vi "StateMachineRealTimeTrackerVI.vi"() -> ()   [LabVIEW 2015]
uses:
  StateMachineObjectTracker/qsm/type defs/mode buttons.ctl
  StateMachineObjectTracker/qsm/type defs/state.ctl
  StateMachineObjectTracker/qsm/type defs/data.ctl
  StateMachineObjectTracker/qsm/type defs/task.ctl
  <vilib>/myRIO/Instrument Drivers/Onboard IO/DIO/typedefs/DIO Reference.ctl
  <vilib>/myRIO/Common/Instrument Driver Framework/Utilities/typedefs/myRIO Generic Hardware Reference.ctl
  <vilib>/myRIO/Common/Instrument Driver Framework/Utilities/typedefs/Hardware Version Enum.ctl
  <vilib>/myRIO/Common/Instrument Driver Framework/Utilities/typedefs/myRIO v1.0 Reference.ctl
  <vilib>/myRIO/Common/Instrument Driver Framework/Utilities/typedefs/Generic FPGA Reference.ctl
  <vilib>/myRIO/Common/Instrument Driver Framework/myRIO v1.0/DIO/typedefs/DIO Channels List.ctl
  <vilib>/myRIO/Common/Instrument Driver Framework/myRIO v1.0/DIO/typedefs/DIO Channels Enum.ctl
  <vilib>/userdefined/High Color/nirio_resource_hc.ctl
  <vilib>/myRIO/Common/Instrument Driver Framework/Utilities/vis/Is FPGA Ref Available.vi
  <vilib>/myRIO/Common/Instrument Driver Framework/myRIO v1.0/DIO/vis/myRIO v1.1 Open DIO.vi
  <vilib>/myRIO/Instrument Drivers/Onboard IO/DIO/vis/Write.vi
  <vilib>/myRIO/Common/Instrument Driver Framework/Utilities/vis/Validate Channels.vi
  <vilib>/myRIO/Common/Instrument Driver Framework/myRIO v1.0/DIO/vis/myRIO v1.0 Reserve DIO.vi
  <vilib>/myRIO/Common/Instrument Driver Framework/myRIO v1.0/Resource Manager/vis/myRIO v1.0 Reserve Channel List.vi
  <vilib>/myRIO/Common/Instrument Driver Framework/myRIO v1.0/DIO/vis/myRIO v1.0 Build MUX Configuration DIO.vi
  <vilib>/myRIO/Common/Instrument Driver Framework/myRIO v1.0/Resource Manager/vis/myRIO v1.0 Reserve Channel.vi
  <vilib>/myRIO/Common/Instrument Driver Framework/myRIO v1.0/Resource Manager/vis/myRIO v1.0 Unreserve Channel.vi
  <vilib>/myRIO/Common/Instrument Driver Framework/myRIO v1.0/Resource Manager/vis/myRIO v1.0 Create Configuration List.vi
  <vilib>/myRIO/Common/Instrument Driver Framework/myRIO v1.0/Resource Manager/vis/myRIO v1.0 Build Mutex Name.vi
  <vilib>/Utility/VariantDataType/GetNumericInfo.vi
  <vilib>/Utility/error.llb/Error Cluster From Error Code.vi
  <vilib>/myRIO/Common/Instrument Driver Framework/myRIO v1.0/myRIO v1.1 Open.vi
  <vilib>/myRIO/Common/Instrument Driver Framework/Utilities/vis/IO Manager.vi
  <vilib>/myRIO/Common/Instrument Driver Framework/Utilities/vis/Configuration Manager.vi
  <vilib>/myRIO/Common/Instrument Driver Framework/myRIO v1.0/Resource Manager/vis/myRIO v1.0 Configure IO.vi
  <vilib>/myRIO/Common/Instrument Driver Framework/myRIO v1.0/myRIO v1.0 Close.vi
  <vilib>/myRIO/Common/Instrument Driver Framework/myRIO v1.0/DIO/vis/myRIO v1.0 Write DIO.vi
  <vilib>/myRIO/Express VI/Onboard Devices/LED/LED Express VI.xnode
  <vilib>/myRIO/Instrument Drivers/Onboard IO/DIO/vis/myRIO DIO Open.xnode
  <vilib>/myRIO/Instrument Drivers/Onboard IO/DIO/DIO.lvlib
panel:
  in  "Stop":bool
  in  "mode buttons":T1
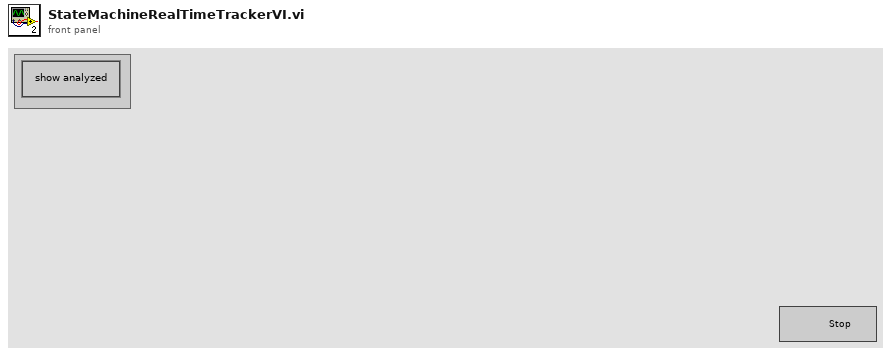
[diagram p1: front panel]
types:
  T1 = typedef "mode buttons.ctl" = cluster{"show analyzed":bool}
  T2 = typedef "data.ctl" = cluster{"Status Test":string}
  T3 = typedef "state.ctl" = enum16{"(qsm) schedule", "(qsm) initialize", "(qsm) release", "(qsm) clean up", "(qsm) shutdown", "(myRIO) initialize", "(myRIO) clean up", "(myRIO) update ports", "(image) get", "(image) analyze", "(image) overlay", "(image) show", "save image", "state A", "state B", "state C", "state D", "state E", "state F", "state G", "state H"}
  T4 = typedef "DIO.lvlib/DIO Reference.ctl" = cluster{"myRIO Reference":T5, "DIO Channels List":T9}
  T5 = typedef "myRIO Generic Hardware Reference.ctl" = cluster{"myRIO Model":T6, "myRIO Hardware Reference":T7}
  T6 = typedef "Hardware Version Enum.ctl" = enum16{"Unknown", "myRIO-1900", "myRIO-1950", "roboRIO"}
  T7 = typedef "myRIO v1.0 Reference.ctl" = cluster{"Generic FPGA Reference":T8, "Allow multiple opens":bool}
  T8 = typedef "Generic FPGA Reference.ctl" = refnum<k20>
  T9 = typedef "DIO Channels List.ctl" = T10[]
  T10 = typedef "DIO Channels Enum.ctl" = enum16{"Not Connected", "C/DIO0", "C/DIO1", "C/DIO2", "C/DIO3", "C/DIO4", "C/DIO5", "C/DIO6", "C/DIO7", "A/DIO0", "A/DIO1", "A/DIO2", "A/DIO3", "A/DIO4", "A/DIO5", "A/DIO6", "A/DIO7", "A/DIO8", "A/DIO9", "A/DIO10", "A/DIO11", "A/DIO12", "A/DIO13", "A/DIO14", "A/DIO15", "B/DIO0", "B/DIO1", "B/DIO2", "B/DIO3", "B/DIO4", "B/DIO5", "B/DIO6", "B/DIO7", "B/DIO8", "B/DIO9", "B/DIO10", "B/DIO11", "B/DIO12", "B/DIO13", "B/DIO14", "B/DIO15", "LED0", "LED1", "LED2", "LED3", "Button0", "DIO/DIO0", "DIO/DIO1", "DIO/DIO2", "DIO/DIO3", "DIO/DIO4", "DIO/DIO5", "DIO/DIO6", "DIO/DIO7", "DIO/DIO8", "DIO/DIO9", "SPI/CS0", "SPI/CS1", "SPI/CS2", "SPI/CS3", "LED RADIO (Green)", "LED RADIO (Red)", "LED COMM (Green)", "LED COMM (Red)", "LED MODE (Green)", "LED MODE (Red)"}
  T11 = typedef "nirio_resource_hc.ctl" = tag
  T12 = typedef "task.ctl" = T3[]
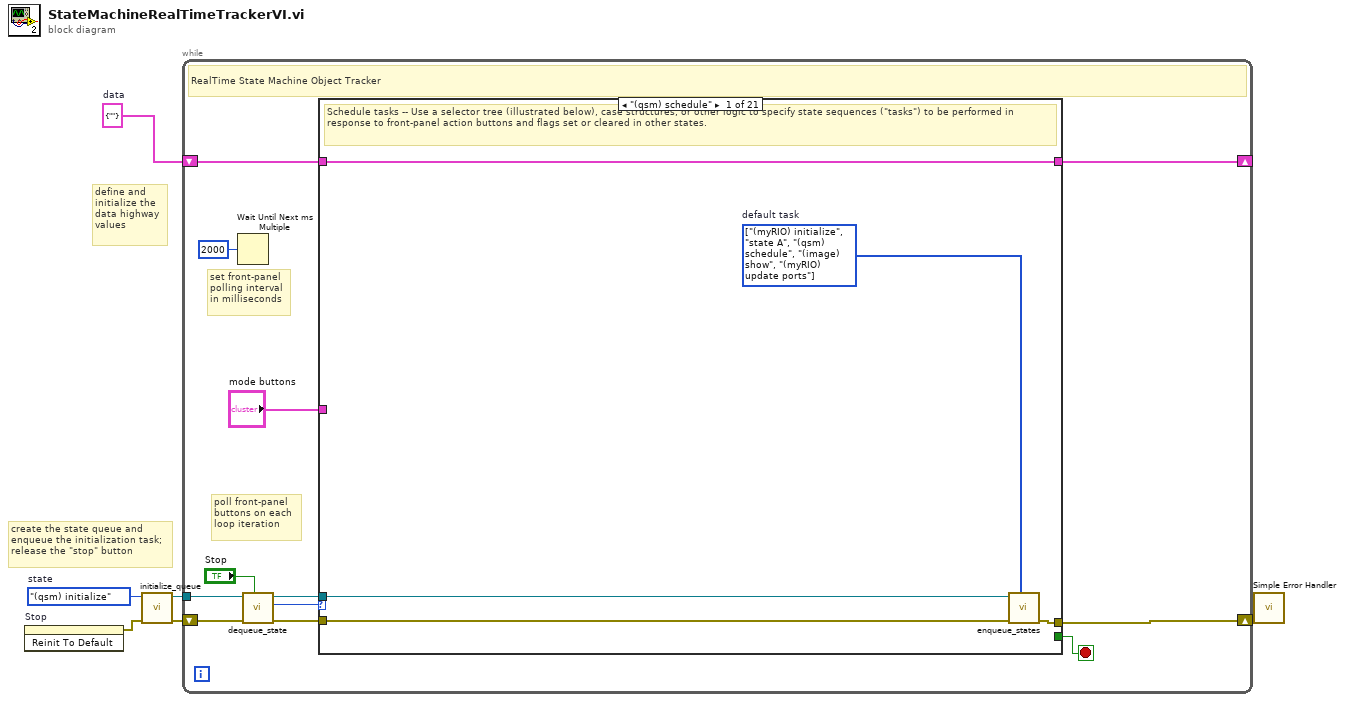
[diagram p0: block diagram]
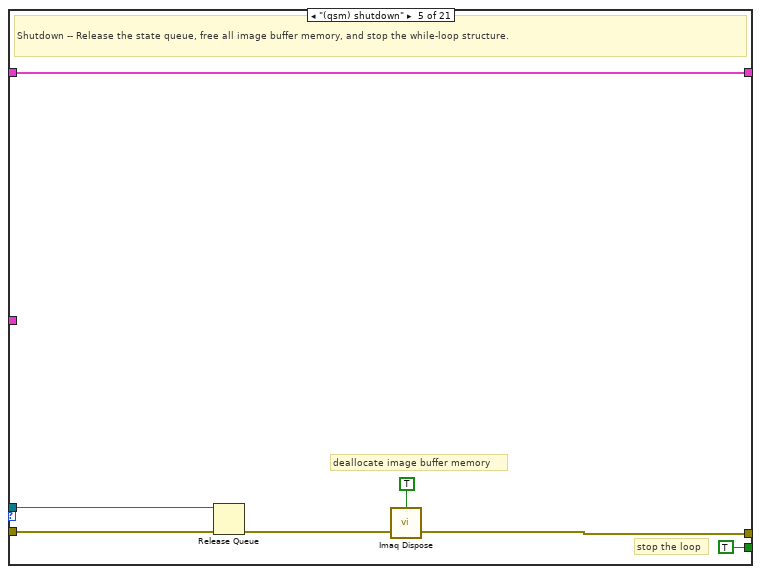
[diagram p5: hidden frame]
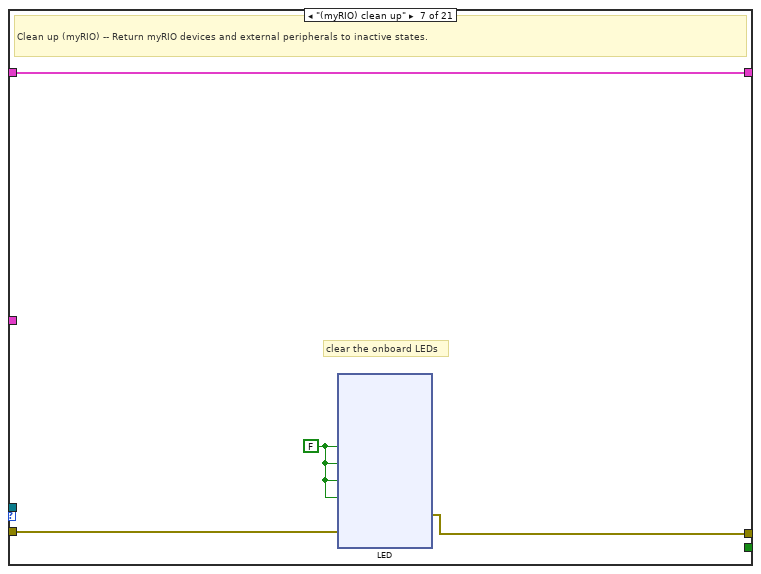
[diagram p7: hidden frame]
diagram:
  w5 = T2 {"Status Test"=""}  # data
  w1 = state."(qsm) initialize"  # state
  # "define and \ninitialize the \ndata highway\nvalues"
  # "create the state queue and\nenqueue the initialization task;\nrelease the \"stop\" button"
  n1 = invoke on="Stop" class="Bool" method="Reinit To Default"() -> (error out=w2:errorcluster)  [unwired: 3 in, 2 out]
  n2 = call "initialize_queue.vi"("error in (no error)"=w2, "state"=w1) -> ("error out"=w4:errorcluster, "queue out"=w3:refnum<queue>)  [unwired: 8 in]
  n3 = while {
    shift-right: [w18] -> w6
    shift-left: w4 -> [w12]
    tunnel: w3 -> [w13]
    shift-right: [w16] -> _
    shift-left: w5 -> [w17]
    stop <- w15 stop-if-true
    # "set front-panel\npolling interval\nin milliseconds"
    # "poll front-panel\nbuttons on each\nloop iteration"
    # "RealTime State Machine Object Tracker"
    n4 = Wait Until Next ms Multiple(millisecond multiple=u32 2000) -> ()  [unwired: 1 out]
    n5 = call "dequeue_state.vi"("stop"="Stop", "error in (no error)"=w12, "queue in"=w13) -> ("error out"=w14:errorcluster, "state"=w7:T3, "queue out"=w10:refnum<queue>)  [unwired: 6 in]
    n6 = case shown="\"(qsm) schedule\"" w7 {
      tunnel: w14 -> [w20 w25 w26 w29 w35 w37 w40 w82 w83 w85 w87 w89 w92 w94 w96 w98 w100 w102 w103 w105 w108]
      tunnel: w10 -> [w21 _ _ _ w34 _ _ _ _ _ _ _ _ _ _ _ _ _ _ _ _]
      tunnel: [w22 w25 w26 w29 w30 w37 w39 w82 w83 w85 w87 w89 w92 w94 w96 w98 w100 w102 w103 w105 w108] -> w18
      tunnel: w17 -> [w23 w24 w27 w28 w33 w38 w42 w81 w84 w86 w88 w90 w91 w93 w95 w97 w99 w101 w104 w106 w107]
      tunnel: [w23 w24 w27 w28 w33 w38 w42 w81 w84 w86 w88 w90 w91 w93 w95 w97 w99 w101 w104 w106 w107] -> w16
      tunnel: [_ _ _ _ TRUE _ _ _ _ _ _ _ _ _ _ _ _ _ _ _ _] -> w15
      tunnel: "mode buttons" -> [_ _ _ _ _ _ _ _ _ _ _ _ _ _ _ _ _ _ _ _ _]
      frame "(qsm) schedule" {
        w19 = T12 [enum."(myRIO) initialize", enum."state A", enum."(qsm) schedule", enum."(image) show", enum."(myRIO) update ports"] items=["(qsm) schedule", "(qsm) initialize", "(qsm) release", "(qsm) clean up", "(qsm) shutdown", "(myRIO) initialize", "(myRIO) clean up", "(myRIO) update ports", "(image) get", "(image) analyze", "(image) overlay", "(image) show", "save image", "state A", "state B", "state C", "state D", "state E", "state F", "state G", "state H"]  # default task
        # "Schedule tasks -- Use a selector tree (illustrated below), case structures, or other logic to specify state sequences (\"tasks\") to be performed in response to front-panel action buttons and flags set or cleared in other states."
        n7 = call "enqueue_states.vi"("task"=w19, "error in"=w20, "queue in"=w21) -> ("error out"=w22:errorcluster)  [unwired: 7 in, 1 out]
      }
      frame "(qsm) initialize" {
        # "Initialize -- Allocate memory for additional image buffers, if necessary, and perform other one-time initialization steps."
      }
      frame "(qsm) release" {
        # "Release all front-panel action buttons."
      }
      frame "(qsm) clean up" {
        # "Clean up -- Set the \"Stop webcam flag\" and perform other necessary clean-up actions."
      }
      frame "(qsm) shutdown" {
        # "deallocate image buffer memory"
        # "stop the loop"
        # "Shutdown -- Release the state queue, free all image buffer memory, and stop the while-loop structure."
        n8 = Release Queue(queue=w34, error in (no error)=w35) -> (error out=w31:errorcluster)  [unwired: 1 in, 2 out]
        n9 = call "Imaq Dispose"("All Images? (No)"=TRUE, "error in (no error)"=w31) -> ("error out"=w30:errorcluster)  [unwired: 4 in]
      }
      frame "(myRIO) initialize" {
        # "Initialize (myRIO) -- Open channels, configure devices, send setup strings to peripherals, etc."
      }
      frame "(myRIO) clean up" {
        w41 = FALSE ("LED3")
        # "clear the onboard LEDs"
        # "Clean up (myRIO) -- Return myRIO devices and external peripherals to inactive states."
        n10 = xnode "LED"("LED0"=w41, "LED1"=w41, "LED2"=w41, "LED3"=w41, "error in (no error)"=w40) -> ("error out"=w39:errorcluster)
      }
      frame "(myRIO) update ports" {
        # "Update ports (myRIO) -- Read and write onboard devices and external peripherals."
      }
      frame "(image) get" {
        # "Get image -- Retrieve a single webcam image frame and optionally flip the image right side up."
      }
      frame "(image) analyze" {
        # "Analyze image -- Analyze the webcam image with a Vision Assistant script."
      }
      frame "(image) overlay" {
        # "Add overlay -- insert a nondestructive data information overlay into the main image display."
      }
      frame "(image) show" {
        # "Show image -- Select from among the available image buffers to show on the main image display; use a selector tree or case structure."
      }
      frame "save image" {
        # "Save image (example of an application-specific state) -- Save either the original webcam image or the analyzed image with overlay to a PNG file on the USB flash drive connected to myRIO."
      }
      frame "state A" {
        # "Expansion State A"
      }
      frame "state B" {
        # "Expansion State B"
      }
      frame "state C" {
        # "Expansion State C"
      }
      frame "state D" {
        # "Expansion State D"
      }
      frame "state E" {
        # "Expansion State E"
      }
      frame "state F" {
        # "Expansion State F"
      }
      frame "state G" {
        # "Expansion State G"
      }
      frame "state H" {
        # "Expansion State H"
      }
    }
  }
  n11 = call <vilib>:"Simple Error Handler.vi"("error in (no error)"=w6) -> ()  [unwired: 4 in, 5 out]
